vi "Source CSM.vi"() -> ()   [LabVIEW 2017]
doc: "Template for building CSM Module without User Interface.\n\n<b>Inputs:</b>\n- <b>Name (\"\" to Use UUID)</b>: Module Name\n - If Input is \"\", an uuid will be used for module name. The module is marked as stand-alone mode and will not be included in module list.\n - Fi Input end with '#', the module will worked in worker mode. Modules with the same name will shared the same message queue. Any external message will be processed by one of the modules, depends on who is free.\n - Otherwise, the input string will be used as module name, which should be unique in system. CSM will go to \"Critical Error\" state if duplicated module name is used in system.\n\n<b>Outputs:</b>\n - N/A"
uses:
  src/user.lib/_NEVSTOP/Communicable State Machine(CSM)/AdvanceAPI/CSM - Revert Arguments-Safe String.vi
  src/user.lib/_NEVSTOP/Communicable State Machine(CSM)/AdvanceAPI/CSM - Break Down Multiple States String.vi
  src/user.lib/_NEVSTOP/Communicable State Machine(CSM)/AdvanceAPI/CSM - Compact Multiple States.vi
  src/user.lib/_NEVSTOP/Communicable State Machine(CSM)/AdvanceAPI/CSM - Make String Arguments Safe.vi
  src/user.lib/_NEVSTOP/Communicable State Machine(CSM)/_Support/Common/Format Timestamp.vi
  src/user.lib/_NEVSTOP/Communicable State Machine(CSM)/AdvanceAPI/CSM - Keywords.vi
  src/user.lib/_NEVSTOP/Communicable State Machine(CSM)/_Shared/Trim Single-line Text.vi
  src/user.lib/_NEVSTOP/Communicable State Machine(CSM)/Communicable State Machine.lvlib
panel:
  out "Error Occurred":errorcluster
  out "State History":string
  in  "Name (\"\" to Use UUID)":string="CSM-Module"
  in  "Init State(\"Macro: Initialize\")":string="Macro: Initialize"
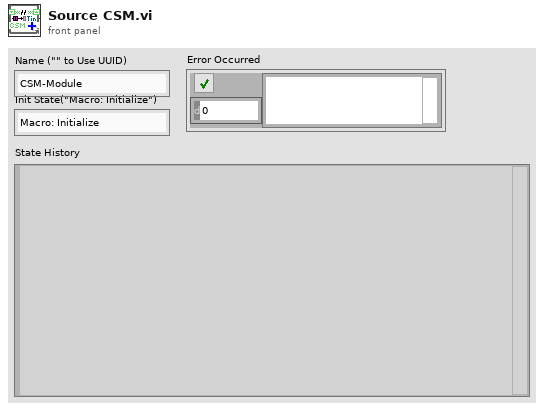
[diagram p1: front panel]
types:
  T1 = enum32{"Invalid", "Standard", "Closed", "Hidden", "Minimized", "Maximized"}
  T2 = enum32{"invalid app kind", "Development System", "Run Time System", "Student Edition", "Embedded LabVIEW", "Evaluation", "Custom"}
  T3 = typedef "Communicable State Machine.lvlib/_CSM_Response Source Message.ctl" = cluster{"‘State":string, "’Arguments":string, "’Error":errorcluster}
  T4 = cluster{"Core":cluster{"Current VI Reference":refnum<vi>, "Close Panel on Exit?":bool}, "Your Boolean data":bool, "Your string data":string}
  T5 = cluster{"Current VI Reference":refnum<vi>, "Close Panel on Exit?":bool}
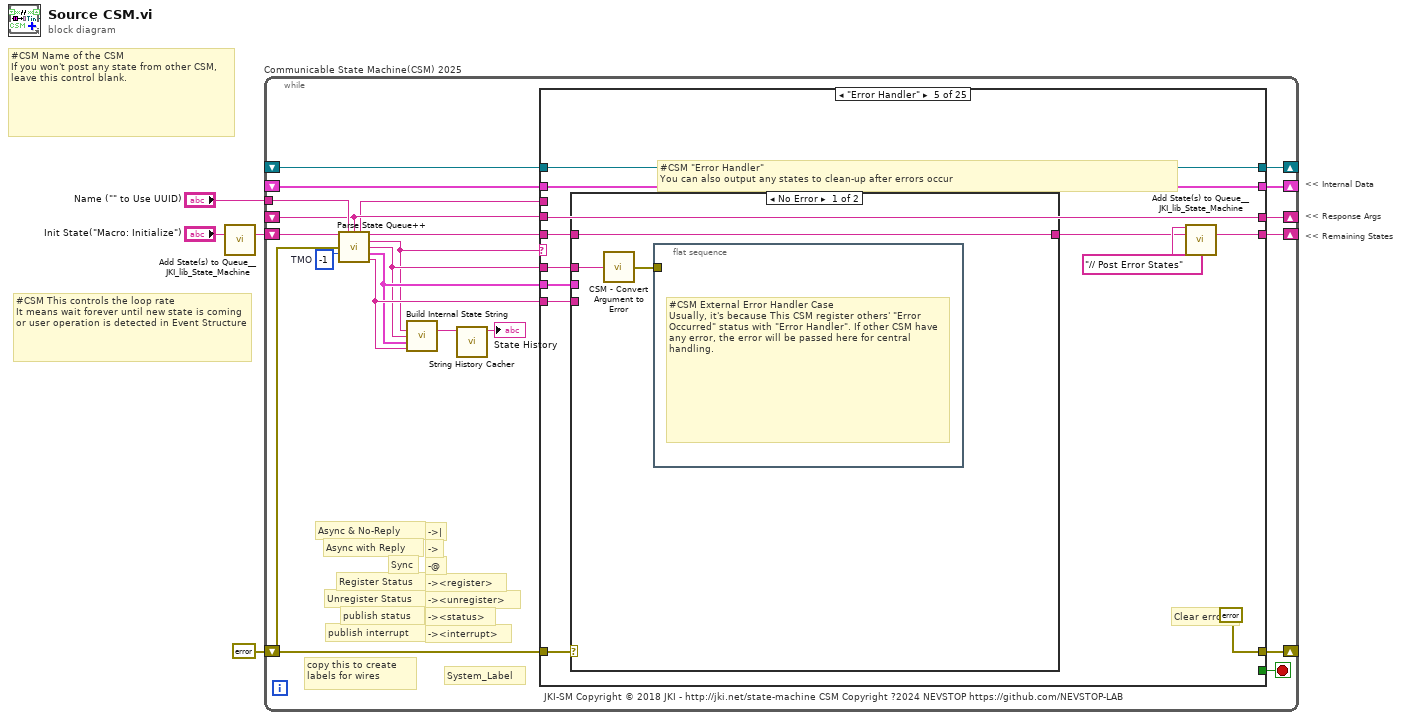
[diagram p0: block diagram]
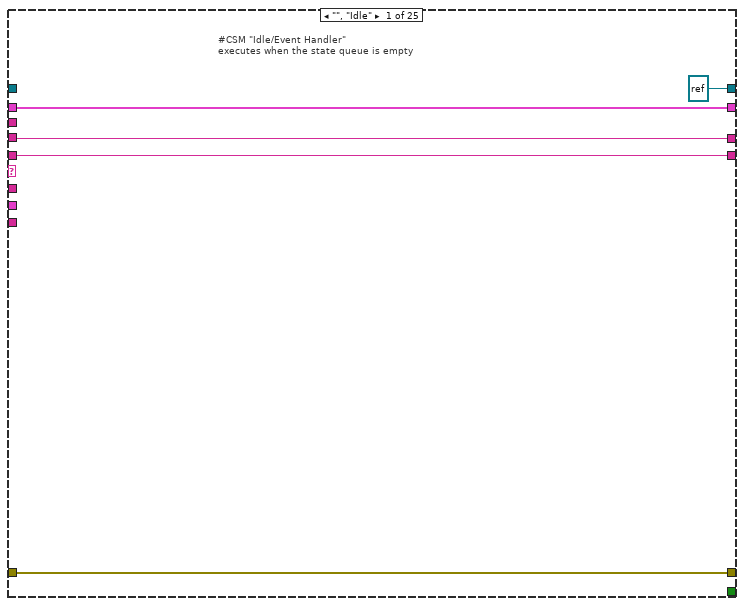
[diagram p2: hidden frame]
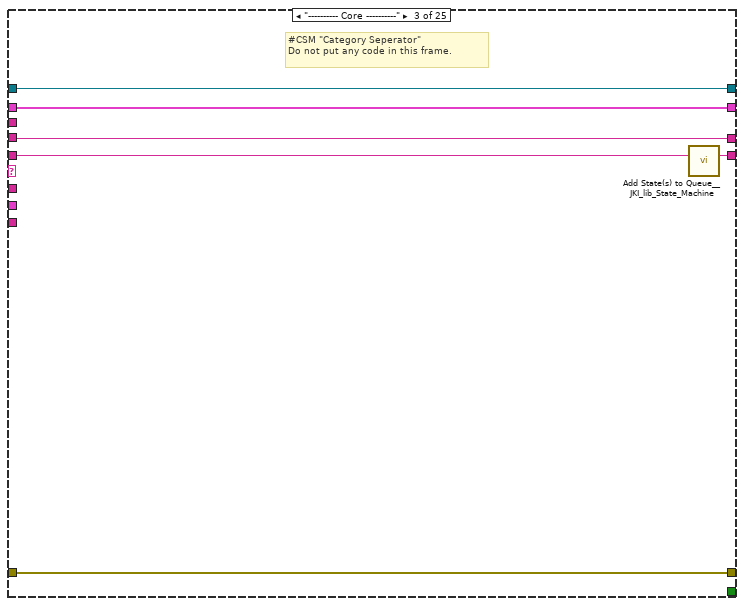
[diagram p4: hidden frame]
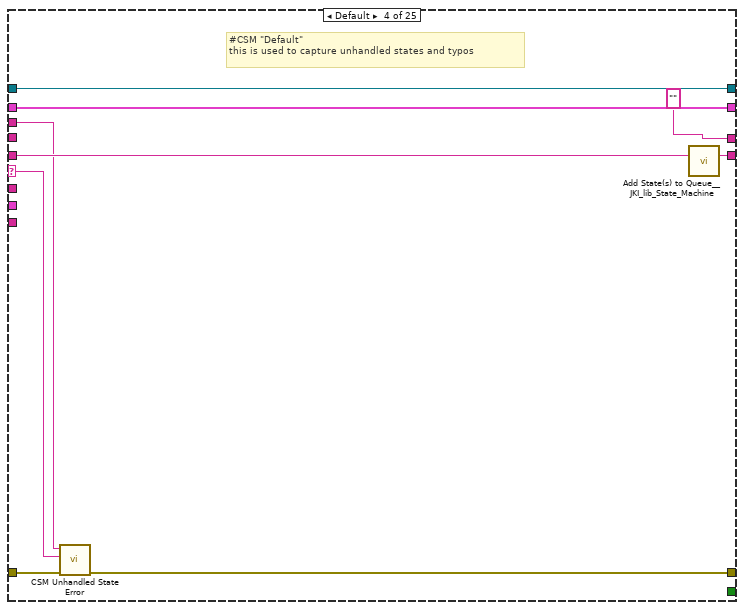
[diagram p5: hidden frame]
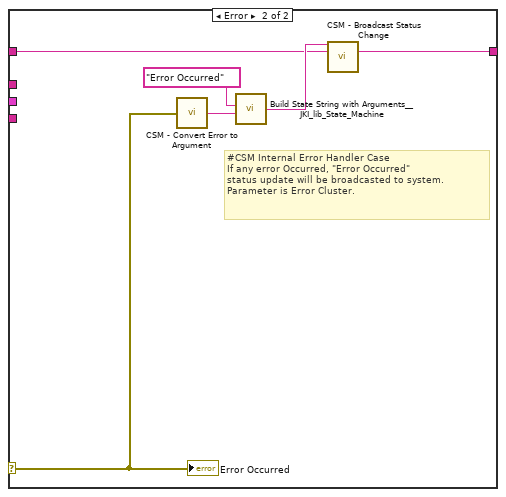
[diagram p6: hidden frame]
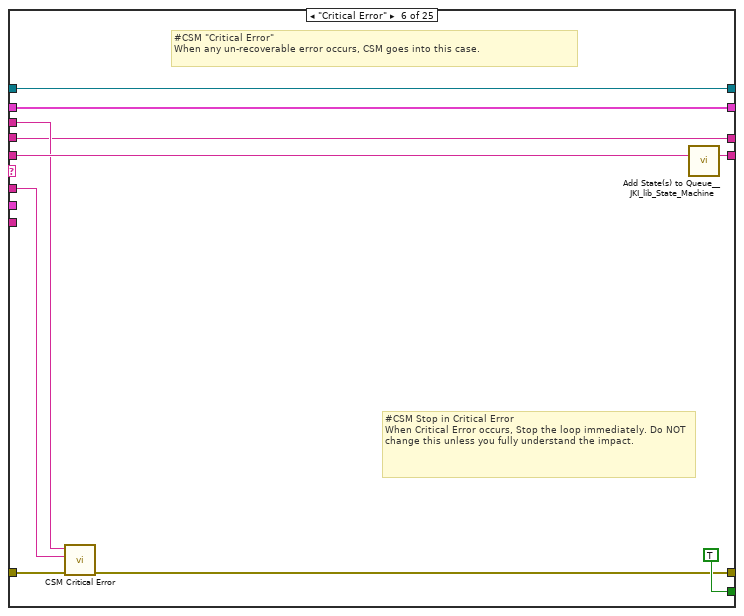
[diagram p7: hidden frame]
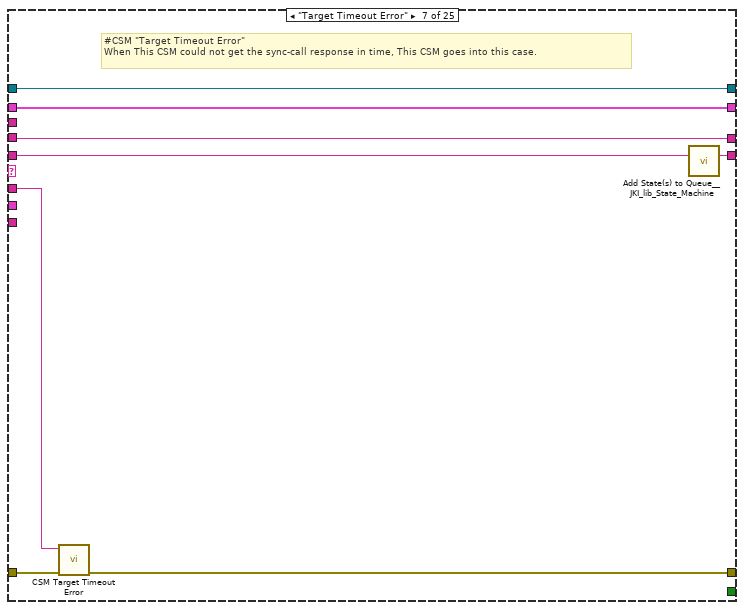
[diagram p8: hidden frame]
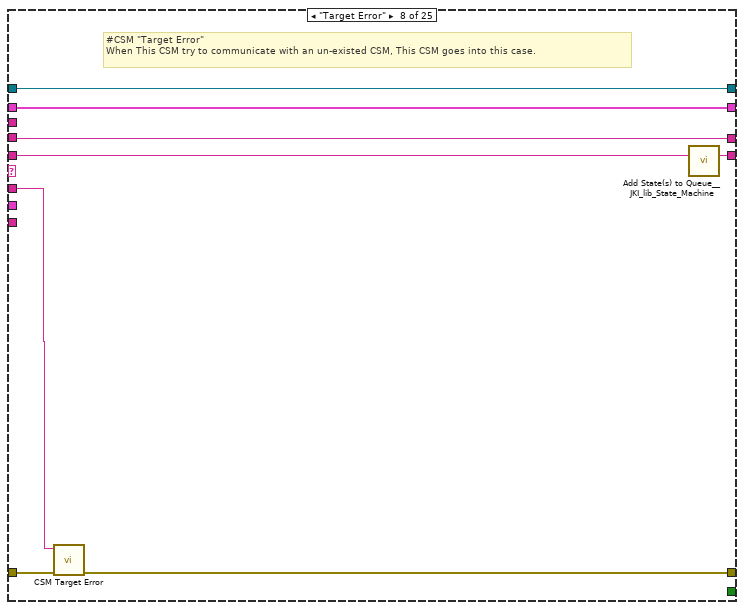
[diagram p9: hidden frame]
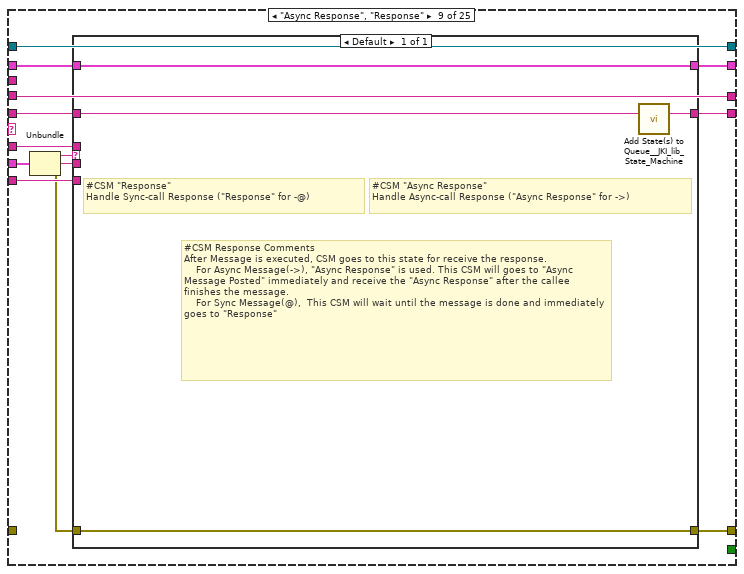
[diagram p10: hidden frame]
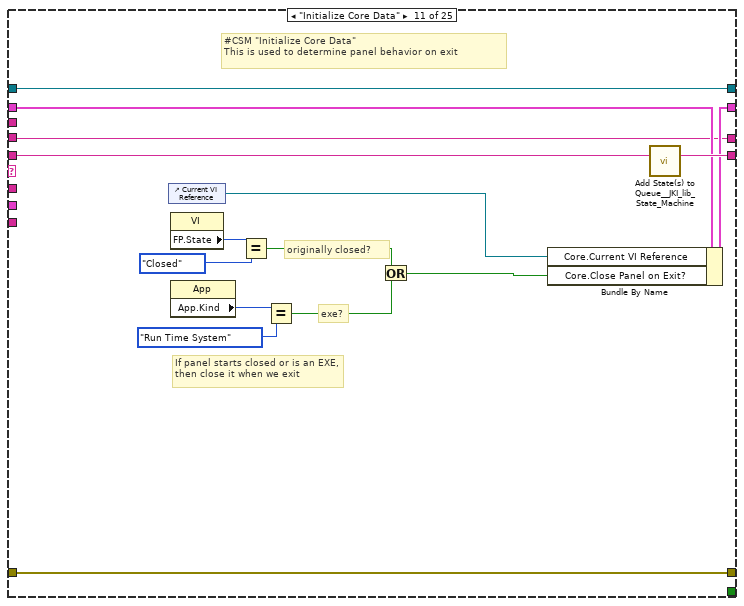
[diagram p12: hidden frame]
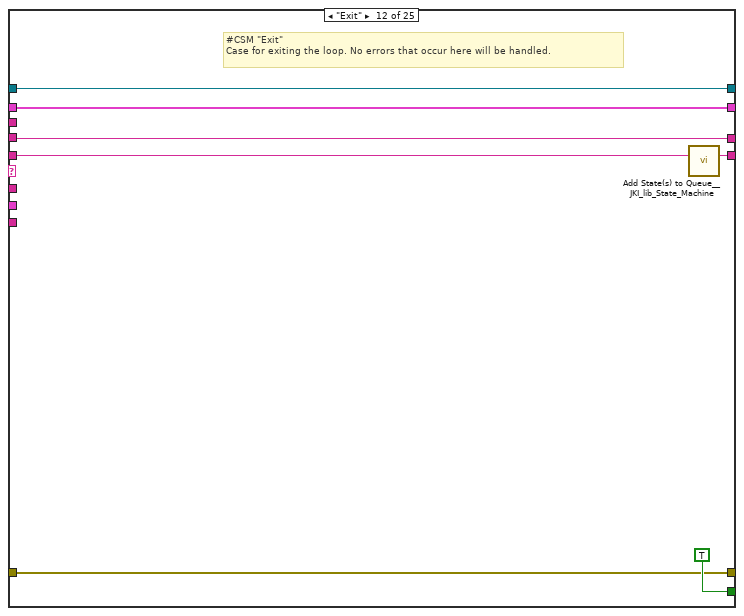
[diagram p13: hidden frame]
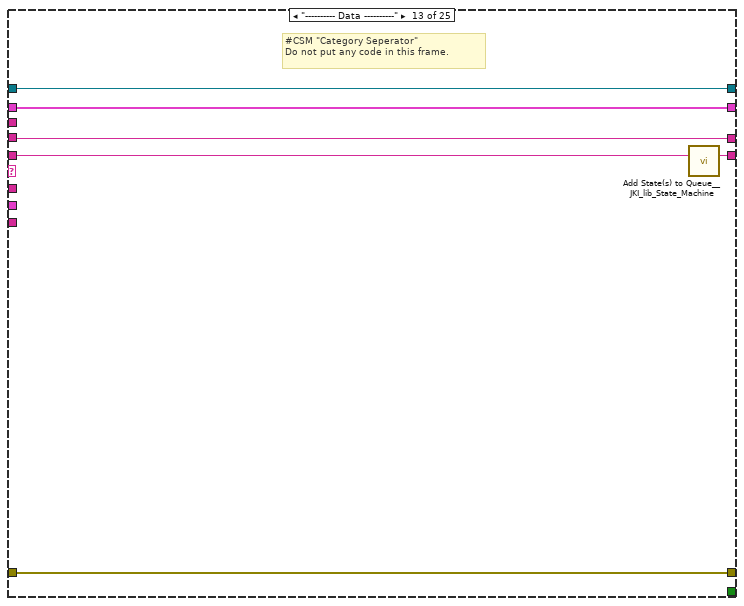
[diagram p14: hidden frame]
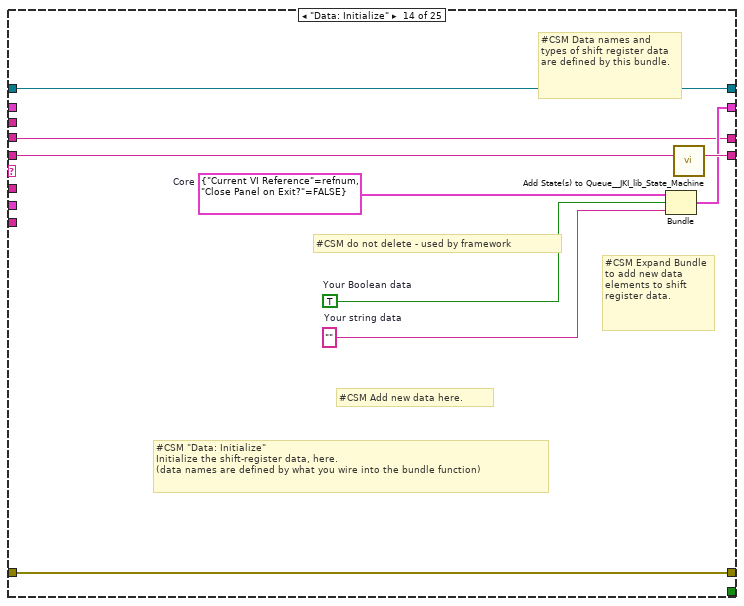
[diagram p15: hidden frame]
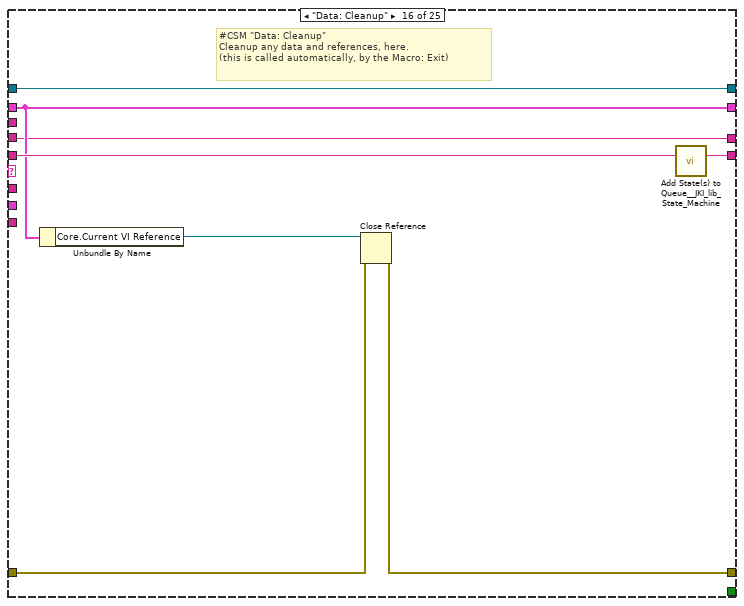
[diagram p17: hidden frame]
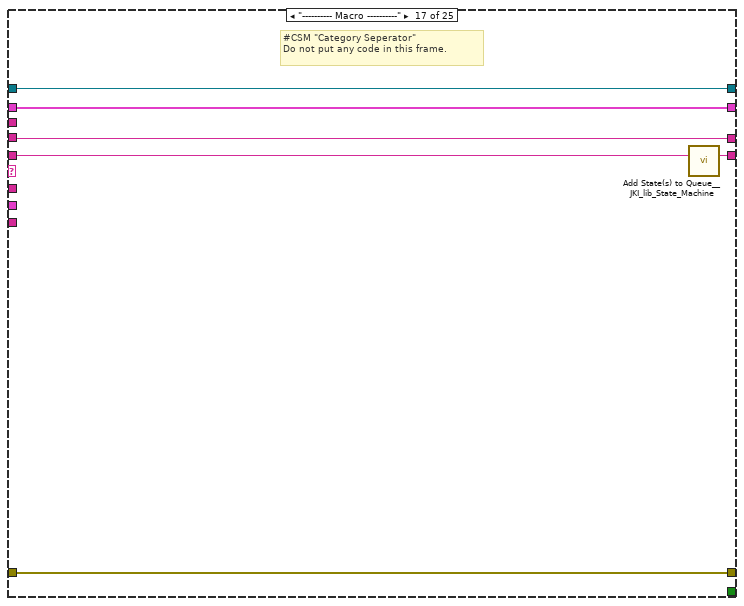
[diagram p18: hidden frame]
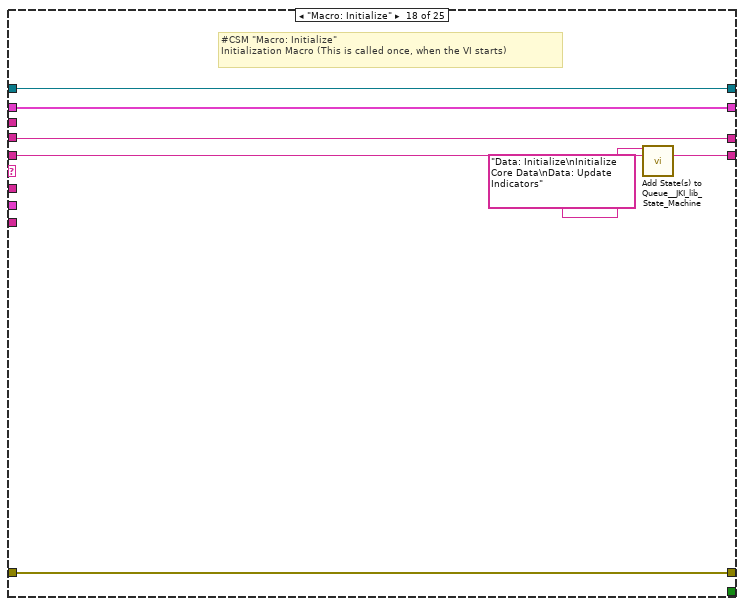
[diagram p19: hidden frame]
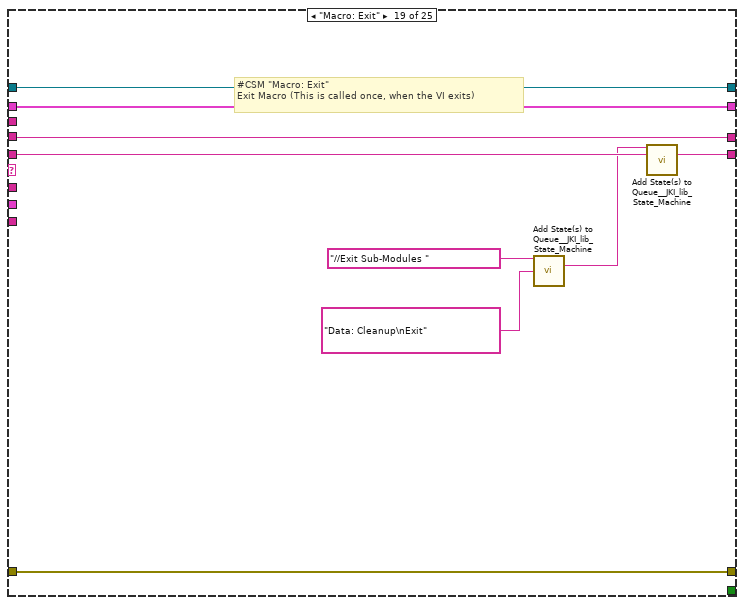
[diagram p20: hidden frame]
diagram:
  # "#CSM Name of the CSM\nIf you won't post any state from other CSM, leave this control blank."
  # "#CSM This controls the loop rate\nIt means wait forever until new state is coming or user operation is detected in Event Structure"
  # "<< Internal Data"
  # "<< Response Args"
  # "<< Remaining States"
  n1 = call <vilib>:"Add State(s) to Queue__JKI_lib_State_Machine.vi"("State(s) in (\"\")"="Init State(\"Macro: Initialize\")") -> ("States Out"=w1:string)  [unwired: 14 in]
  n2 = while "Communicable State Machine(CSM) 2025" {
    shift-right: [w20] -> _
    shift-left: _ -> [w19]
    shift-right: [w23] -> _
    shift-left: errorcluster {"status"=FALSE, "code"=0, "source"=""} ("error out") -> [w9]
    shift-right: [w22] -> _
    shift-left: w1 -> [w24]
    tunnel: "Name (\"\" to Use UUID)" -> [w16]
    shift-right: [w17] -> _
    shift-left: _ -> [w11]
    shift-right: [w8] -> _
    shift-left: _ -> [w7]
    stop <- w21 stop-if-true
    w18 = -1  # TMO
    # "-><interrupt>"
    # "-><status>"
    # "-><unregister>"
    # "-><register>"
    # "-@"
    # "->"
    # "->|"
    # "publish interrupt"
    # "publish status"
    # "Unregister Status"
    # "Register Status"
    # "Sync"
    # "Async with Reply"
    # "Async & No-Reply"
    # "JKI-SM Copyright © 2018 JKI - http://jki.net/state-machine CSM Copyright ?2024 NEVSTOP https://github.com/NEVSTOP-LAB"
    # "copy this to create labels for wires"
    # "System_Label"
    n3 = call "Parse State Queue++.vi"("State Queue"=w24, "Name (\"\" to Use UUID)"=w16, "Response Arguments"=w11, "Previous Error"=w9, "Dequeue (1 ms)"=w18) -> ("Name Used"=w10:string, "Remaining States"=w25:string, "Current State"=w12:string, "Arguments"=w13:string, "Additional Information"=w14:T3, "Source CSM"=w15:string)  [unwired: 5 in]
    n4 = call "Build Internal State String.vi"("State"=w12, "Arguments (\"\")"=w13, "Additional Information"=w14, "Source (\"\")"=w15) -> ("State With Arguments"=w6:string)  [unwired: 11 in]
    n5 = call "String History Cacher.vi"("String"=w6) -> ("String Cache"=→"State History":string)  [unwired: 10 in]
    n6 = case shown="\"Error Handler\"" w12 {
      selector: w12 -> [_ _ _ w45 _ _ _ _ _ _ _ _ _ _ _ _ _ _ _ _ _ _ _ _ _]
      tunnel: w25 -> [w30 w34 w40 w49 w55 w80 w88 w96 w108 w118 w133 w140 w146 w155 w160 w168 w174 w181 w190 w195 w200 w206 w214 w220 w226]
      tunnel: w13 -> [_ _ _ _ w54 w76 w85 w93 w102 _ _ _ _ _ _ _ _ _ _ _ _ w204 _ _ _]
      tunnel: w19 -> [w29 w31 w38 w47 w60 w78 w86 w94 w106 w117 w127 w138 w144 _ w159 w163 w172 w179 w188 w194 w199 w205 w212 w218 w224]
      tunnel: [w28 w33 w37 w42 errorcluster {"status"=FALSE, "code"=0, "source"=""} ("error out") w73 w83 w91 w109 w116 w121 w136 w143 w149 w158 w164 w171 w177 w184 w193 w197 w202 w211 w217 w223] -> w23
      tunnel: w9 -> [w28 w33 w37 w43 w58 w74 w84 w92 _ w116 w121 w136 w143 w149 w158 w165 w171 w177 w184 w193 w197 w202 w211 w217 w223]
      tunnel: [w30 w34 w39 w48 w56 w79 w87 w95 w107 w118 w132 w139 w145 w154 w160 w167 w173 w180 w189 w195 w200 w206 w213 w219 w225] -> w22
      tunnel: [_ _ _ _ _ TRUE _ _ _ _ _ TRUE _ _ _ _ _ _ _ _ _ _ _ _ _] -> w21
      tunnel: [w29 w31 w38 w47 w60 w78 w86 w94 w105 w117 w131 w138 w144 w153 w159 w163 w172 w179 w188 w194 w199 w205 w212 w218 w224] -> w20
      tunnel: w15 -> [_ _ _ _ w51 _ _ _ w103 _ _ _ _ _ _ _ _ _ _ _ _ _ _ _ _]
      tunnel: w14 -> [_ _ _ _ w52 _ _ _ w104 _ _ _ _ _ _ _ _ _ _ _ _ _ _ _ _]
      tunnel: [w27 _ w36 "" w53 w72 w82 w90 w98 w115 w120 w135 w142 w148 w157 w162 w170 w176 w183 w192 "API1 Response" w203 w210 w216 w222] -> w17
      tunnel: w10 -> [_ _ _ w44 _ w75 _ _ _ _ _ _ _ _ _ _ _ _ _ _ _ _ _ _ _]
      tunnel: w11 -> [w27 _ w36 _ w53 w72 w82 w90 w98 w115 w120 w135 w142 w148 w157 w162 w170 w176 w183 w192 _ _ w210 w216 w222]
      tunnel: [refnum<file> refnum ("refnum out") w32 w35 w41 w50 w71 w81 w89 w97 w114 w119 w134 w141 w147 w156 w161 w169 w175 w182 w191 w196 w201 w209 w215 w221] -> w8
      tunnel: w7 -> [_ w32 w35 w41 w50 w71 w81 w89 w97 w114 w119 w134 w141 w147 w156 w161 w169 w175 w182 w191 w196 w201 w209 w215 w221]
      frame "", "Idle" {
        # "#CSM \"Idle/Event Handler\"\nexecutes when the state queue is empty"
      }
      frame "CSM Documentation" {
        # "#CSM Documentation"
        # "#CSM State Syntax\n\n// Comment line, all text to the right of “//” will be ignored\n// Local Message Example\nDoSth: DoA >> Arguments\n\n// Sync Call Example\nAPI: xxxx >> Arguments -@ TargetModule\n\n// Async Call Example\nAPI: xxxx >> Arguments -> TargetModule\n\n// Async Call without Reply Example\nAPI: xxxx >> Arguments ->| TargetModule\n\n// Broadcast normal status:\nStatus >> StatusArguments  -><status>\n\n// Broadcast Interrupt status:\nInterrupt >> StatusArguments  -><interrupt>\n\n// Register Source Module's status to Handler Module\nStatus@Source Module >> Handler Module@Handler Module -><register>\n\n// Unegister Source Module's status\nStatus@Source Module >> Handler Module -><unregister>"
        # "#CSM README FIRST\n\nCommunicable State Machine(CSM) is a LabVIEW application framework that builds upon JKI State Machine(JKISM). It follows the pattern of JKISM and extends the keywords to describe message communication between modules, including concepts such as Sync-Message, Async-Message, Subscription/Unsubscription of status - essential elements for creating reusable code modules. For more information, please visit the CSM wiki: https://nevstop-lab.github.io/CSM-Wiki/\n\nFor instructions on JKI State Machine, visit: \n    http://jki.net/state-machine/\nFor information about CSM, visit: \n    https://github.com/NEVSTOP-LAB"
        # "#CSM \"Documentation\"\nCase for holding CSM Documenation"
      }
      frame "---------- Core ----------" {
        # "#CSM \"Category Seperator\"\nDo not put any code in this frame."
        n7 = call <vilib>:"Add State(s) to Queue__JKI_lib_State_Machine.vi"("State(s) in (\"\")"=w40) -> ("States Out"=w39:string)  [unwired: 14 in]
      }
      frame Default {
        # "#CSM \"Default\"\nthis is used to capture unhandled states and typos"
        n8 = call "CSM Unhandled State Error.vi"("error in (no error)"=w43, "Undefined State"=w45, "CSM Name"=w44) -> ("error out"=w42:errorcluster)  [unwired: 8 in]
        n9 = call <vilib>:"Add State(s) to Queue__JKI_lib_State_Machine.vi"("State(s) in (\"\")"=w49) -> ("States Out"=w48:string)  [unwired: 14 in]
      }
      frame "Error Handler" {
        # "#CSM \"Error Handler\"\nYou can also output any states to clean-up after errors occur"
        # "Clear error"
        n10 = case shown="No Error" w58 {
          selector: w58 -> [_ w65]
          tunnel: [w64 w67] -> w57
          tunnel: w55 -> [w64 w66]
          tunnel: w54 -> [w63 _]
          tunnel: w52 -> [_ _]
          tunnel: w51 -> [_ _]
          frame No Error {
            n11 = call "CSM - Convert Argument to Error.vi"("Argument"=w63) -> ("Error"=w62:errorcluster)  [unwired: 4 in]
            n12 = flat-sequence {
              tunnel: w62 -> [_]
              frame #0 {
                # "#CSM External Error Handler Case\nUsually, it's because This CSM register others' \"Error Occurred\" status with \"Error Handler\". If other CSM have any error, the error will be passed here for central handling."
              }
            }
          }
          frame Error {
            # "#CSM Internal Error Handler Case \nIf any error Occurred, \"Error Occurred\" \nstatus update will be broadcasted to system.\nParameter is Error Cluster."
            n13 = call "CSM - Convert Error to Argument.vi"("Error"=w65) -> ("Argument"=w69:string)  [unwired: 4 in]
            n14 = call <vilib>:"Build State String with Arguments__JKI_lib_State_Machine.vi"("Arguments (\"\")"=w69, "State"="Error Occurred" ("Status with Arguments")) -> ("State with Arguments"=w68:string)  [unwired: 4 in]
            n15 = call "CSM - Broadcast Status Change.vi"("Status With Arguments"=w68, "State Queue"=w66) -> ("Remaining States"=w67:string)  [unwired: 13 in]
            "Error Occurred" <- w65
          }
        }
        n16 = call <vilib>:"Add State(s) to Queue__JKI_lib_State_Machine.vi"("State(s) in Front (\"\")"="// Post Error States", "State(s) in (\"\")"=w57) -> ("States Out"=w56:string)  [unwired: 13 in]
      }
      frame "Critical Error" {
        # "#CSM \"Critical Error\"\nWhen any un-recoverable error occurs, CSM goes into this case."
        # "#CSM Stop in Critical Error\nWhen Critical Error occurs, Stop the loop immediately. Do NOT change this unless you fully understand the impact."
        n17 = call "CSM Critical Error.vi"("error in (no error)"=w74, "Arugments (As Reason)"=w76, "CSM Name"=w75) -> ("error out"=w73:errorcluster)  [unwired: 8 in]
        n18 = call <vilib>:"Add State(s) to Queue__JKI_lib_State_Machine.vi"("State(s) in (\"\")"=w80) -> ("States Out"=w79:string)  [unwired: 14 in]
      }
      frame "Target Timeout Error" {
        # "#CSM \"Target Timeout Error\"\nWhen This CSM could not get the sync-call response in time, This CSM goes into this case."
        n19 = call "CSM Target Timeout Error.vi"("error in (no error)"=w84, "Arguments (As CSM Name)"=w85) -> ("error out"=w83:errorcluster)  [unwired: 9 in]
        n20 = call <vilib>:"Add State(s) to Queue__JKI_lib_State_Machine.vi"("State(s) in (\"\")"=w88) -> ("States Out"=w87:string)  [unwired: 14 in]
      }
      frame "Target Error" {
        # "#CSM \"Target Error\"\nWhen This CSM try to communicate with an un-existed CSM, This CSM goes into this case."
        n21 = call "CSM Target Error.vi"("error in (no error)"=w92, "Arguments (As CSM Name)"=w93) -> ("error out"=w91:errorcluster)  [unwired: 9 in]
        n22 = call <vilib>:"Add State(s) to Queue__JKI_lib_State_Machine.vi"("State(s) in (\"\")"=w96) -> ("States Out"=w95:string)  [unwired: 14 in]
      }
      frame "Async Response", "Response" {
        n23 = Unbundle(w104) -> ("‘State"=w101:string, "’Arguments"=w100:string, "’Error"=w99:errorcluster)
        n24 = case shown="Default" w101 {
          tunnel: [w110] -> w107
          tunnel: w108 -> [w111]
          tunnel: [w113] -> w105
          tunnel: w106 -> [w113]
          tunnel: [w112] -> w109
          tunnel: w99 -> [w112]
          tunnel: w103 -> [_]
          tunnel: w102 -> [_]
          tunnel: w100 -> [_]
          frame Default {
            # "#CSM \"Async Response\"\nHandle Async-call Response (\"Async Response\" for ->)"
            # "#CSM \"Response\"\nHandle Sync-call Response (\"Response\" for -@)"
            # "#CSM Response Comments\nAfter Message is executed, CSM goes to this state for receive the response.\n    For Async Message(->), \"Async Response\" is used. This CSM will goes to \"Async Message Posted\" immediately and receive the \"Async Response\" after the callee finishes the message.\n    For Sync Message(@),  This CSM will wait until the message is done and immediately goes to \"Response\""
            n25 = call <vilib>:"Add State(s) to Queue__JKI_lib_State_Machine.vi"("State(s) in (\"\")"=w111) -> ("States Out"=w110:string)  [unwired: 14 in]
          }
        }
      }
      frame "Async Message Posted" {
        # "#CSM \"Async Message Posted\"\nAfter Async Message is posted (-> or ->| ), CSM goes to this state for post-action.\nYou can use Argument - State to tell which Async Message is called."
      }
      frame "Initialize Core Data" {
        # "#CSM \"Initialize Core Data\"\nThis is used to determine panel behavior on exit"
        # "originally closed?"
        # "exe?"
        # "If panel starts closed or is an EXE, then close it when we exit"
        n26 = control-ref of="Current VI Reference"() -> (w125:refnum<vi>)
        n27 = property class="VI"() -> ("FP.State"=w124:T1)  [unwired: 2 in, 2 out]
        n28 = property class="App"() -> ("App.Kind"=w130:T2)  [unwired: 2 in, 2 out]
        n29 = Equal?(x=w124, y=T1."Closed" ("Front Panel Window:State")) -> (x = y?=w122:bool)
        n30 = Equal?(x=w130, y=T2."Run Time System" ("Application:Kind")) -> (x = y?=w128:bool)
        n31 = Or(x=w122, y=w128) -> (x .or. y?=w126:bool)
        n32 = Bundle By Name(cluster=w127, "Core.Current VI Reference"=w125, "Core.Close Panel on Exit?"=w126) -> (w131:T4)
        n33 = call <vilib>:"Add State(s) to Queue__JKI_lib_State_Machine.vi"("State(s) in (\"\")"=w133) -> ("States Out"=w132:string)  [unwired: 14 in]
      }
      frame "Exit" {
        # "#CSM \"Exit\"\nCase for exiting the loop. No errors that occur here will be handled."
        n34 = call <vilib>:"Add State(s) to Queue__JKI_lib_State_Machine.vi"("State(s) in (\"\")"=w140) -> ("States Out"=w139:string)  [unwired: 14 in]
      }
      frame "---------- Data ----------" {
        # "#CSM \"Category Seperator\"\nDo not put any code in this frame."
        n35 = call <vilib>:"Add State(s) to Queue__JKI_lib_State_Machine.vi"("State(s) in (\"\")"=w146) -> ("States Out"=w145:string)  [unwired: 14 in]
      }
      frame "Data: Initialize" {
        w150 = T5 {"Current VI Reference"=refnum, "Close Panel on Exit?"=FALSE}  # Core
        w152 = TRUE  # Your Boolean data
        w151 = ""  # Your string data
        # "#CSM \"Data: Initialize\"\nInitialize the shift-register data, here.\n(data names are defined by what you wire into the bundle function)"
        # "#CSM do not delete - used by framework"
        # "#CSM Expand Bundle to add new data elements to shift register data."
        # "#CSM Add new data here."
        # "#CSM Data names and types of shift register data are defined by this bundle."
        n36 = Bundle("Core"=w150, "Your Boolean data"=w152, "Your string data"=w151) -> (w153:T4)  [unwired: 1 in]
        n37 = call <vilib>:"Add State(s) to Queue__JKI_lib_State_Machine.vi"("State(s) in (\"\")"=w155) -> ("States Out"=w154:string)  [unwired: 14 in]
      }
      frame "Data: Update Indicators" {
      }
      frame "Data: Cleanup" {
        # "#CSM \"Data: Cleanup\"\nCleanup any data and references, here.\n(this is called automatically, by the Macro: Exit)"
        n38 = Unbundle By Name(w163) -> ("Core.Current VI Reference"=w166:refnum<vi>)
        n39 = Close Reference(reference=w166, error in (no error)=w165) -> (error out=w164:errorcluster)
        n40 = call <vilib>:"Add State(s) to Queue__JKI_lib_State_Machine.vi"("State(s) in (\"\")"=w168) -> ("States Out"=w167:string)  [unwired: 14 in]
      }
      frame "---------- Macro ----------" {
        # "#CSM \"Category Seperator\"\nDo not put any code in this frame."
        n41 = call <vilib>:"Add State(s) to Queue__JKI_lib_State_Machine.vi"("State(s) in (\"\")"=w174) -> ("States Out"=w173:string)  [unwired: 14 in]
      }
      frame "Macro: Initialize" {
        # "#CSM \"Macro: Initialize\"\nInitialization Macro (This is called once, when the VI starts)"
        n42 = call <vilib>:"Add State(s) to Queue__JKI_lib_State_Machine.vi"("State(s) in Front (\"\")"="Data: Initialize\nInitialize Core Data\nData: Update Indicators", "State(s) in (\"\")"=w181) -> ("States Out"=w180:string)  [unwired: 13 in]
      }
      frame "Macro: Exit" {
        # "#CSM \"Macro: Exit\"\nExit Macro (This is called once, when the VI exits)"
        n43 = call <vilib>:"Add State(s) to Queue__JKI_lib_State_Machine.vi"("State(s) in Front (\"\")"="//Exit Sub-Modules ", "State(s) at Back (\"\")"="Data: Cleanup\nExit") -> ("States Out"=w186:string)  [unwired: 13 in]
        n44 = call <vilib>:"Add State(s) to Queue__JKI_lib_State_Machine.vi"("State(s) in Front (\"\")"=w186, "State(s) in (\"\")"=w190) -> ("States Out"=w189:string)  [unwired: 13 in]
      }
      frame "---------- API ----------" {
        # "#CSM \"Category Seperator\"\nDo not put any code in this frame."
      }
      frame "API: API1" {
        # "#CSM API Example\nCopy/Rename this case for your own API"
        # "#CSM >> Msg/Rep's CSM >>\nIf you need to tell who triggered this state , use this string. If it's this case itself, this string is \"\"."
        # "#CSM >> Arguments >>\nDeal with the parameter if any"
        # "#CSM Response\nConnect this to return the response of your API"
      }
      frame "API: API2" {
        # "#CSM API Example\nCopy/Rename this case for your own API"
        # "unpack Hex String  to Variant\nif complex parameter is needed."
        n45 = call "CSM - Convert HexStr to Data.vi"("HEX String"=w204) -> ()  [unwired: 7 in, 2 out]
        n46 = disable-structure shown="Enabled" {
          disable-tunnel: [w207 "API2 Response"] -> w203
          frame Disabled {
            # "pack variant to hexstr \nif complex response is needed."
            # "complex Response"
            n47 = call "CSM - Convert Data to HexStr.vi"() -> ("HEX String (0-9,A-F)"=w207:string)  [unwired: 9 in]
          }
          frame Enabled {
          }
        }
      }
      frame "---------- Action ----------" {
        # "#CSM \"Category Seperator\"\nDo not put any code in this frame."
        n48 = call <vilib>:"Add State(s) to Queue__JKI_lib_State_Machine.vi"("State(s) in (\"\")"=w214) -> ("States Out"=w213:string)  [unwired: 14 in]
      }
      frame "Action: action1" {
        # "#CSM \"Internal State\"\nThis category is used for holding internal states"
        n49 = call <vilib>:"Add State(s) to Queue__JKI_lib_State_Machine.vi"("State(s) in (\"\")"=w220) -> ("States Out"=w219:string)  [unwired: 14 in]
      }
      frame "Action: action2" {
        # "#CSM \"Internal State\"\nThis category is used for holding internal states"
        n50 = call <vilib>:"Add State(s) to Queue__JKI_lib_State_Machine.vi"("State(s) in (\"\")"=w226) -> ("States Out"=w225:string)  [unwired: 14 in]
      }
    }
  }
